vi "I2C_ReadBitFromSlave_2.vi"(8 "error in":errorcluster, 11 "HalfCycle(Ticks)":u32) -> (0 "error out":errorcluster, 3 "Bit":bool)   [LabVIEW 2019]
doc: "Reads a Bit from the Slave Device.\n\nVI Written By:\nPeter Fuller\nSenior Engineer\nplf Consulting, LLC\n617.699.2201"
uses:
  <vilib>/eio/EIONode/EIONode.xnode
  Instance           1 28Saved   I2C_ReadBitFromSlave .vi
  Instance           2 28Saved   I2C_ReadBitFromSlave .vi
  <vilib>/eio/EIOMethodNode/EIOMethodNode.xnode
  <vilib>/rvi/eio/common/nirviEmuTemplateMethod_errors.vi
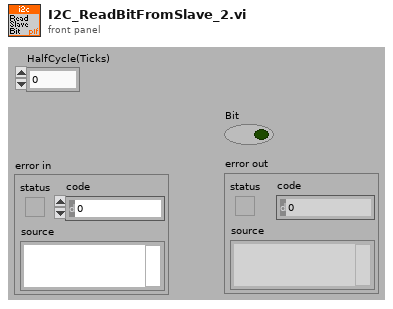
[diagram p1: front panel]
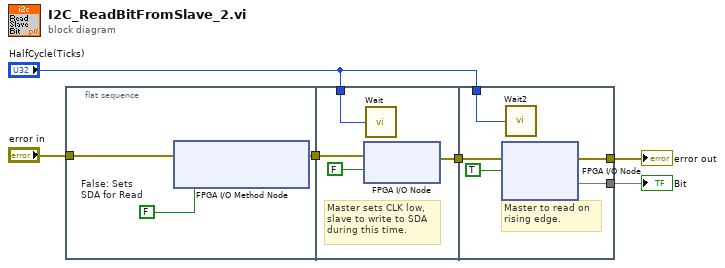
[diagram p0: block diagram]
diagram:
  n1 = flat-sequence {
    tunnel: [w8] -> w4
    tunnel: "error in" -> [w7]
    tunnel: [w11] -> w2
    tunnel: w4 -> [w12]
    tunnel: "HalfCycle(Ticks)" -> [w10]
    tunnel: w2 -> [w16]
    tunnel: "HalfCycle(Ticks)" -> [w14]
    tunnel: [w17] -> w6
    tunnel: [w15] -> w5
    frame #0 {
      w9 = FALSE  # False: Sets  SDA for Read
      n2 = xnode "FPGA I/O Method Node"("error in"=w7, "Enable"=w9) -> ("error out"=w8:errorcluster)  [unwired: 1 in, 1 out]
    }
    frame #1 {
      # "Master sets CLK low, slave to write to SDA during this time."
      n3 = xnode "FPGA I/O Node"("error in"=w12, "SCL2"=FALSE ("Value")) -> ("error out"=w11:errorcluster)  [unwired: 1 in, 1 out]
      n4 = call "Wait"("Count(Ticks)"=w10) -> ()  [unwired: 1 out]
    }
    frame #2 {
      # "Master to read on \nrising edge."
      n5 = xnode "FPGA I/O Node"("error in"=w16, "SCL2"=TRUE ("Value")) -> ("error out"=w15:errorcluster, "SDA2"=w17)  [unwired: 2 in, 2 out]
      n6 = call "Wait2"("Count(Ticks)"=w14) -> ()  [unwired: 1 out]
    }
  }
  "Bit" <- w6
  "error out" <- w5
